vi "ExportFluoFit.vi"(0 "from end?":bool, 3 "time in":dbl[](array[numeric]), 4 "# of lines":i32=32, 5 "lifetimes":dbl[][](array[numeric]), 6 "Lifetime Export Path (ASCII-File)":path) -> ()   [LabVIEW 2009]
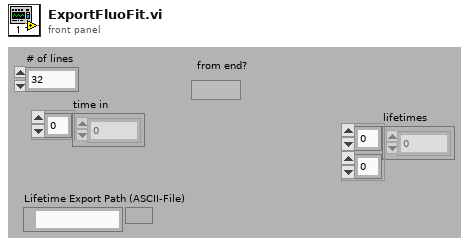
[diagram p1: front panel]
types:
  T1 = typedef "Settings.ctl" = cluster{"threshold":cluster{"max":u32, "min":u32}, "RGB or false color":bool, "16bit":bool, "log/lin axis":u16, "spotsize button":bool, "Pixelsize":u16, "autoscale x":bool, "autoscale y":bool, "correlation":bool, "ADC-Resolution":i32, "F2-lifetime":cluster{"display tau":bool, "display F2":bool, "Palette Number lifetime":enum32{"Gray", "Binary", "Gradient", "Rainbow", "Temperature"}, "Palette Number F2":enum32{"Gray", "Binary", "Gradient", "Rainbow", "Temperature"}, "max tau-Value":dbl, "min tau-Value":dbl, "max F2-Value":dbl, "min F2-Value":dbl}, "TAC-Window 1":u16, "TAC-Window 2":u16, "false color palette":cluster{"1":u32, "2":u32, "3":u32, "4":u32, "5":u32, "6":u32, "7":u32, "8":u32, "8 2":u32, "8 3":u32, "8 4":u32, "8 5":u32}, "rebinning":dbl}
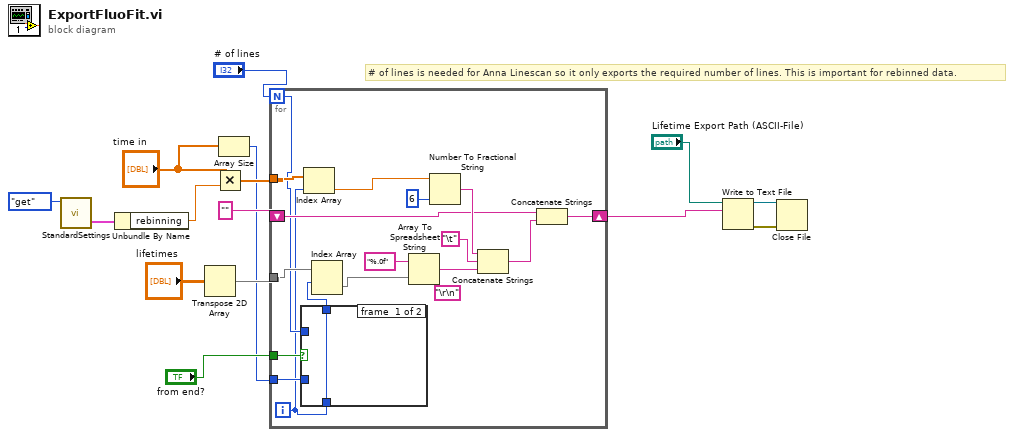
[diagram p0: block diagram]
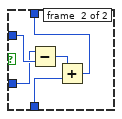
[diagram p2: hidden frame]
diagram:
  # "# of lines is needed for Anna Linescan so it only exports the required number of lines. This is important for rebinned data."
  n1 = call "StandardSettings.vi"("Enum"=enum16{"Load", "get", "Save", "set"}."get") -> ("StandardSettings"=w6:T1)  [unwired: 4 in]
  n2 = Unbundle By Name(w6) -> ("rebinning"=w5:dbl)
  n3 = Transpose 2D Array(2D array="lifetimes") -> (transposed array=w14:dbl[][])
  n4 = Multiply(x="time in", y=w5) -> (x*y=w13:dbl[])
  n5 = Array Size(array="time in") -> (size(s)=w1:i32)
  n6 = for {
    N: "# of lines" -> [w18]
    tunnel: w14 -> [w23]
    tunnel: w13 -> [w24]
    shift-right: [w27] -> w11
    shift-left: "" -> [w26]
    tunnel: "from end?" -> [w20]
    tunnel: w1 -> [w17]
    i -> [w16]
    (unwired) "\r\n"
    n7 = case shown="False" w20 {
      tunnel: [w33 w34] -> w19
      tunnel: w16 -> [w33 w35]
      tunnel: w18 -> [_ w38]
      tunnel: w17 -> [_ w37]
      frame #0 {
      }
      frame #1 {
        n8 = Subtract(x=w37, y=w38) -> (x-y=w36:i32)
        n9 = Add(x=w36, y=w35) -> (x+y=w34:i32)
      }
    }
    n10 = Index Array(array=w24, index=w16) -> (element=w22:dbl)
    n11 = Index Array(array=w23, index (row)=w19) -> (element=w21:dbl[])  [unwired: 1 in]
    n12 = Array To Spreadsheet String(array=w21, 3:"%.0f" ("format (%.3f)")) -> (spreadsheet string=w30:string)  [unwired: 1 in]
    n13 = Number To Fractional String(number=w22, precision (6)=i16 6 ("Genauigkeit (6)")) -> (F-format string=w31:string)  [unwired: 2 in]
    n14 = Concatenate Strings(w31, "\t", w30) -> (w25:string)
    n15 = Concatenate Strings(w26, w25) -> (w27:string)
  }
  n16 = Write to Text File(file (use dialog)="Lifetime Export Path (ASCII-File)", text=w11) -> (refnum out=w9:refnum<file>, error out=w8:errorcluster)  [unwired: 2 in, 1 out]
  n17 = Close File(refnum=w9, error in=w8) -> ()  [unwired: 2 out]
